vi "列表框结合TAB.vi"() -> ()   [LabVIEW 2013]
panel:
  in  "Stop":bool
  out "Title":string
  in  "Select Page":i32(listbox)
  out "选项卡控件":T1(tab)
  out "波形图表":dbl[](graph)
  # "Page2"
  # "Page3"
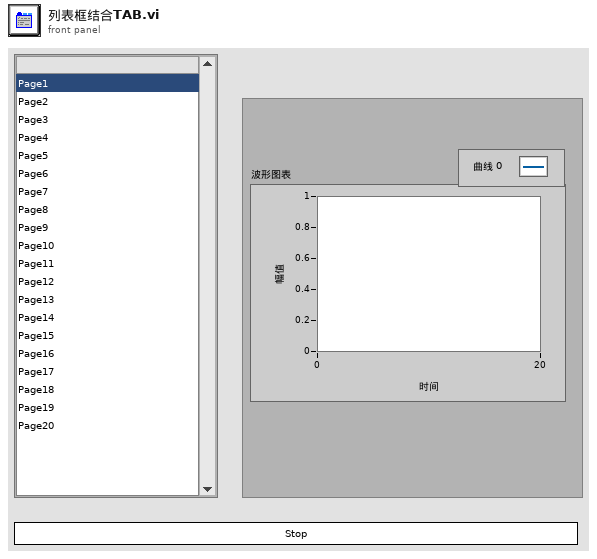
[diagram p1: front panel]
types:
  T1 = enum32{"P1", "P2", "P3", "P4", "P5", "P6", "P7", "P8", "P9", "P10", "P11", "P12", "P13", "P14", "P15", "P16", "P17", "P18", "P19", "P20"}
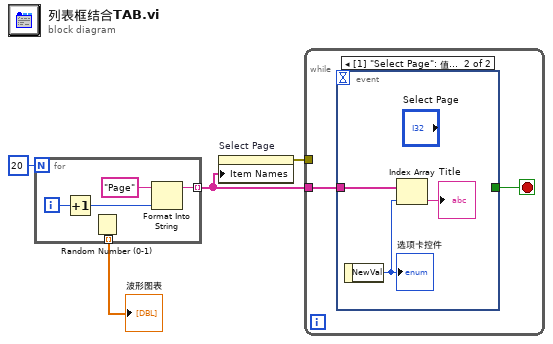
[diagram p0: block diagram]
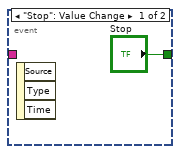
[diagram p2: hidden frame]
diagram:
  n1 = for {
    N: 20 -> [_]
    tunnel: [w6] -> w2 mode=indexing
    tunnel: [w5] -> w1 mode=indexing
    i -> [w9]
    n2 = Increment(x=w9) -> (x+1=w8:i32)
    n3 = Random Number (0-1)() -> (number: 0 to 1=w5:dbl)
    n4 = Format Into String(initial string="Page" ("初始字符串"), w8) -> (resulting string=w6:string)  [unwired: 2 in, 1 out]
  }
  "波形图表" <- w1
  n5 = property on="Select Page" class="LstBox (严格)"("Item Names"=w2) -> (error out=w3:errorcluster)  [unwired: 2 in, 1 out]
  n6 = while {
    tunnel: w3 -> [_]
    tunnel: w2 -> [w10]
    stop <- w11 stop-if-true
    n7 = event shown="[1] \"Select Page\": 值改变" {
      selector: _ -> [_ _]
      dyn-events: _ -> [_ _]
      timeout: _ -> [_ _]
      tunnel: ["Stop" _] -> w11
      tunnel: w10 -> [_ w15]
      event "Stop": Value Change {
        n8 = event-data() -> ()  [unwired: 1 in, 3 out]
      }
      event "Select Page": Value Change {
        n9 = event-data() -> ("NewVal"=w13:i32)  [unwired: 1 in]
        "选项卡控件" <- w13
        n10 = Index Array(array=w15, index=w13) -> (element=→"Title":string)
      }
    }
  }
